vi "Destroy.vi"(0 "reference in":refnum<class "LcWebView.lvclass">, 2 "BlankBrowser(True)":bool=TRUE, 5 "Error In":errorcluster) -> (14 "reference out":refnum<class "LcWebView.lvclass">, 19 "Error Out":errorcluster)   [LabVIEW 2018, in "LcWebView.lvclass"]
uses:
  LcWebView.lvclass
  C:/Projects/LcWebView2/LcWebView/LcWebView_class/data/Microsoft.Web.WebView2.Core.dll
  data/Microsoft.Web.WebView2.Core.dll
  C:/Projects/LcWebView2/LcWebView/LcWebView_class/data/Microsoft.Web.WebView2.WinForms.dll
  data/Microsoft.Web.WebView2.WinForms.dll
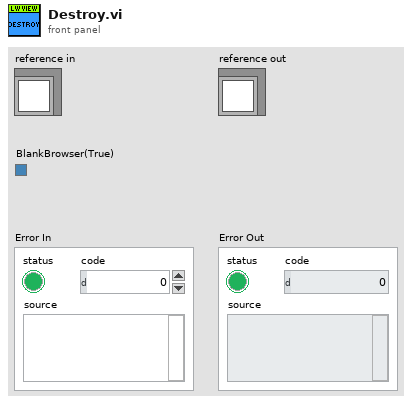
[diagram p1: front panel]
types:
  T1 = typedef "LcWebView.lvclass/ObjectAttributes.ctl" = cluster{"WebView Container":refnum<k24>, "CoreWebViewRef":refnum<k24>, "Status":i32, "Status Message":string, "User Data Folder":path, "BrowserProcessId":u32, "PlotType":T2}
  T2 = typedef "LcWebView.lvclass/PlotType.ctl" = enum16{"bar", "line", "pie", "doughnut", "scatter", "radar", "bubble", "polarArea"}
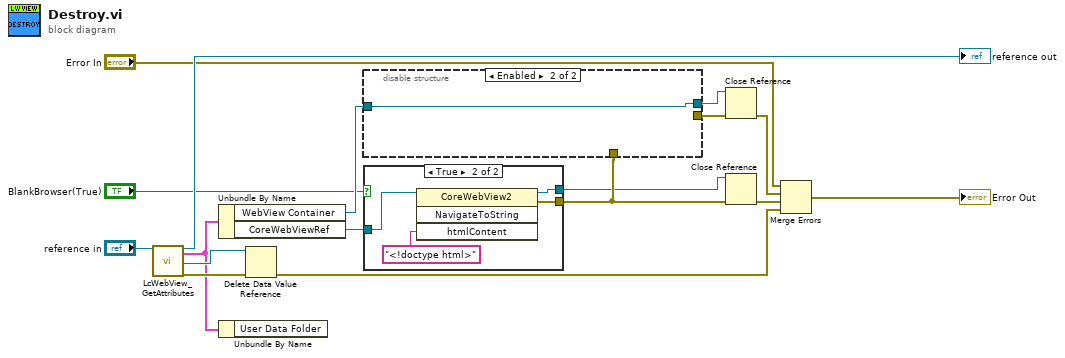
[diagram p0: block diagram]
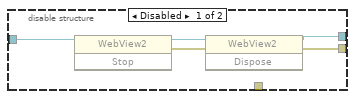
[diagram p3: hidden frame]
diagram:
  n1 = call "LcWebView_GetAttributes.vi"("reference in"="reference in") -> ("reference out"=→"reference out":refnum<class "LcWebView.lvclass">, "Data"=w3:T1, "DataRef"=w14:refnum<data-value>, "error out"=w15:errorcluster)  [unwired: 15 in]
  n2 = Unbundle By Name(w3) -> ("WebView Container"=w12:refnum<k24>, "CoreWebViewRef"=w5:refnum<k24>)
  n3 = Unbundle By Name(w3) -> ()  [unwired: 1 out]
  n4 = Delete Data Value Reference(data value reference=w14, error in=w15) -> (error out=w8:errorcluster)  [unwired: 1 out]
  n5 = case shown="True" "BlankBrowser(True)" {
    tunnel: w5 -> [w18 w22]
    tunnel: [w18 w21] -> w1
    tunnel: [_ w20] -> w2
    frame False {
    }
    frame True {
      n6 = invoke class="CoreWebView2" method="NavigateToString"(reference=w22, "htmlContent"="<!doctype html>") -> (reference out=w21:refnum<k24>, error out=w20:errorcluster)  [unwired: 2 in, 2 out]
    }
  }
  n7 = disable-structure shown="Enabled" {
    disable-tunnel: [w23 _] -> w7
    disable-tunnel: [w24 w28] -> w6
    disable-tunnel: w12 -> [w27 w28]
    disable-tunnel: w2 -> [_ _]
    frame Disabled {
      n8 = invoke class="WebView2" method="Stop"(reference=w27) -> (reference out=w26:refnum<k24>, error out=w25:errorcluster)  [unwired: 2 in, 1 out]
      n9 = invoke class="WebView2" method="Dispose"(reference=w26, error in=w25) -> (reference out=w24:refnum<k24>, error out=w23:errorcluster)  [unwired: 1 in, 1 out]
    }
    frame Enabled {
    }
  }
  n10 = Close Reference(reference=w6, error in (no error)=w7) -> (error out=w13:errorcluster)
  n11 = Close Reference(reference=w1, error in (no error)=w2) -> (error out=w11:errorcluster)
  n12 = Merge Errors("Error In", w13, w11, w8) -> (→"Error Out":errorcluster)
